vi "WPs and Obstacles 4.vi"(8 "Sim Robot Initial Long":dbl, 9 "Sim Robot Initial Lat":dbl, 11 "Real/Sim":bool) -> (0 "Obstacle Lats and Longs":cluster{"Obs Lats":dbl[], "Obs Longs":dbl[]} {"Obs Longs" format="%#_8g"; "Obs Lats" format="%#_8g"}, 1 "WP Lats and Longs":cluster{"WP Lats":dbl[], "WP Longs":dbl[]} {"WP Longs" format="%#_8g"; "WP Lats" format="%#_8g"}, 3 "WP Map":T1(graph))   [LabVIEW 2014]
panel:
  in  "Obstacle Real Longs":dbl[](array[numeric])=[81.2678, 81.267312, 81.267112, 81.267332, 81.267916, 81.267137, 81.267874, 81.267301, 81.267913, 81.26772] format="%#_8g"
  in  "Obstacle Real Lats":dbl[](array[numeric])=[37.1524, 37.152256, 37.152877, 37.152903, 37.152565, 37.152792, 37.152806, 37.152779, 37.152868, 37.152484] format="%#_8g"
  in  "WP Real Longs":dbl[](array[numeric])=[83.1954638, 83.19550076, 81.267112, 81.267332, 81.267916, 81.267137, 81.267874, 81.267301, 81.267913, 81.26772] format="%#_8g"
  in  "WP Real Lats":dbl[](array[numeric])=[42.678172477, 42.677950947, 37.152877, 37.152903, 37.152565, 37.152792, 37.152806, 37.152779, 37.152868, 37.152484] format="%#_8g"
  # "Waypoint and Obstacles 4 (Uses Paint)"
  # "Added Global sim painted map"
  # "Inputs:"
  # "20"
  # "12"
  # "Outputs:"
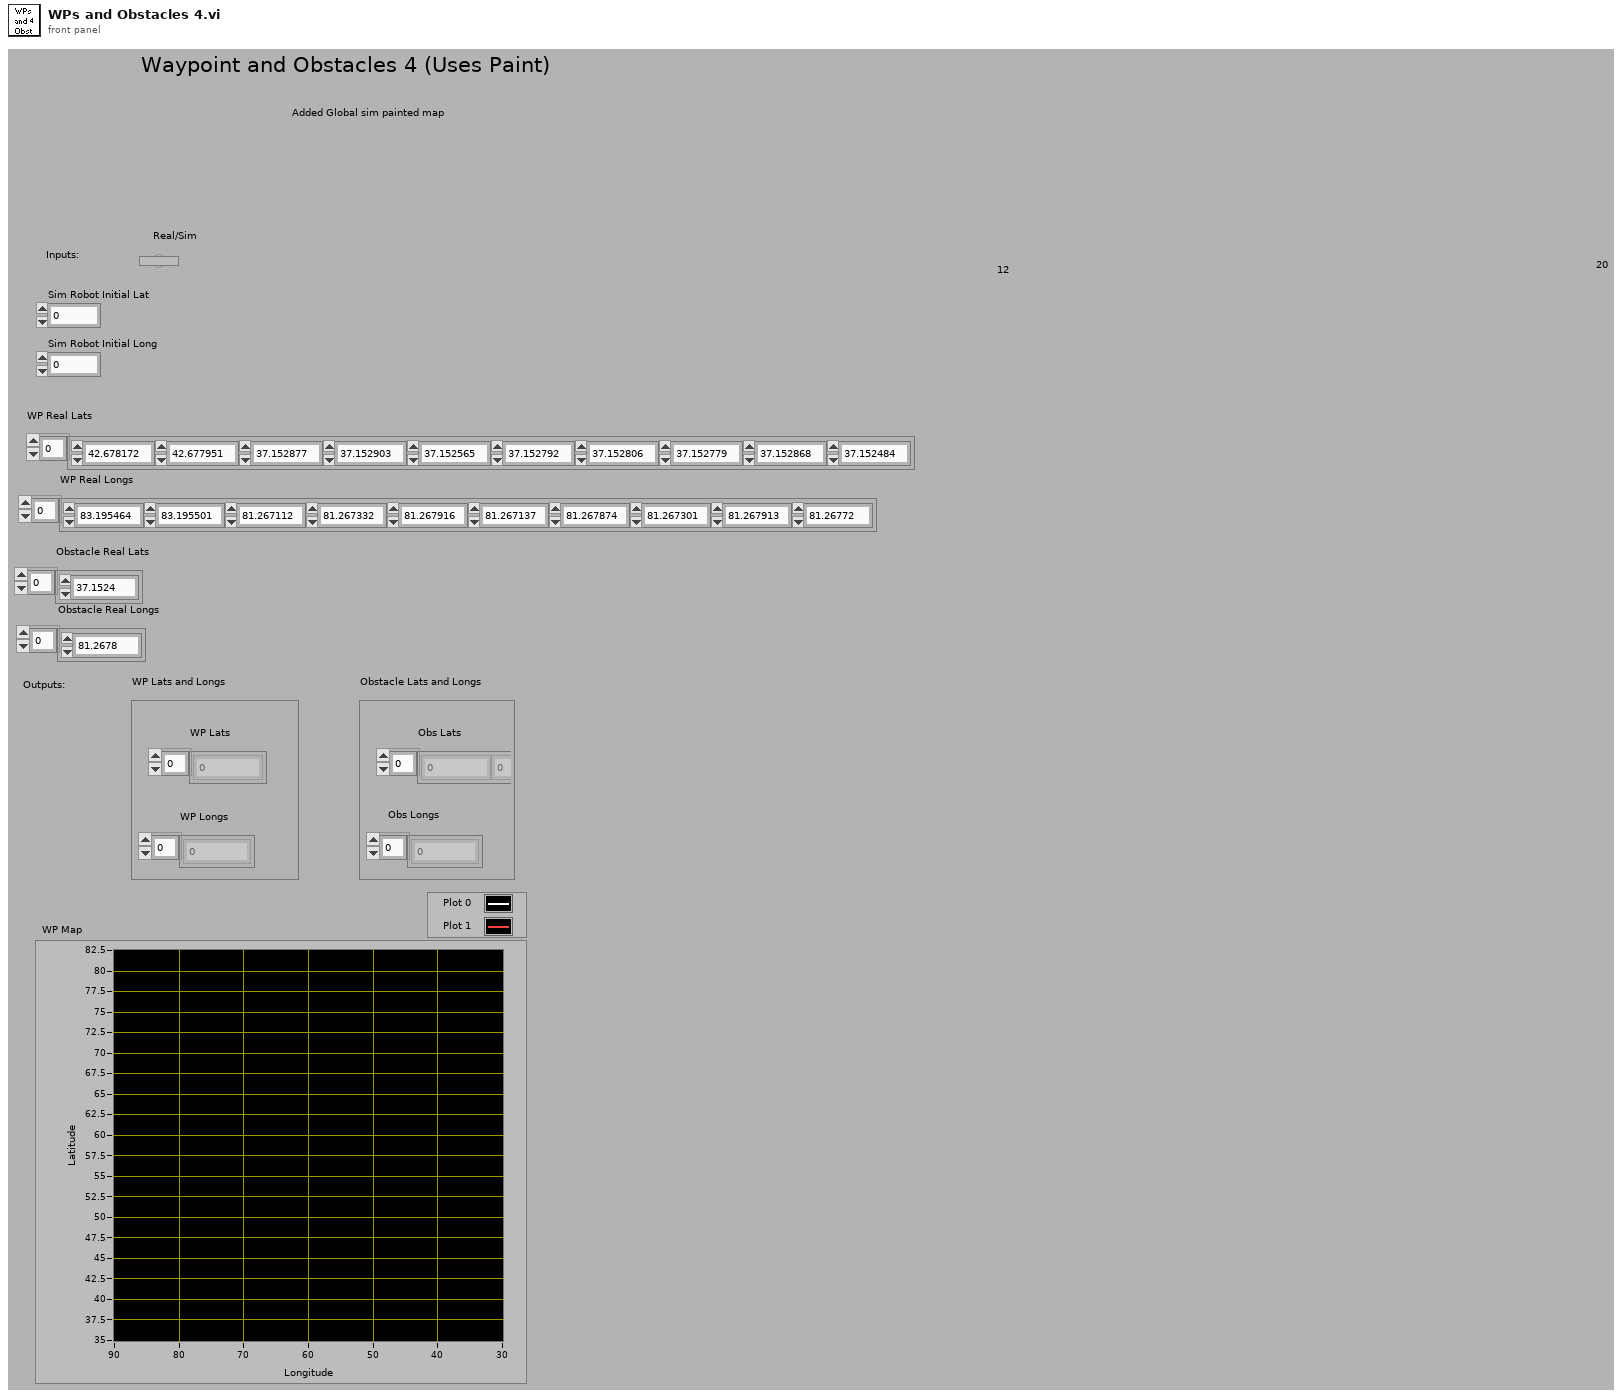
[diagram p1: front panel]
types:
  T1 = cluster{"Obstacle Longs":dbl[], "Obstacle Lats":dbl[]}[]
  T2 = cluster{"Obstacle Longs":dbl[], "Obstacle Lats":dbl[]}
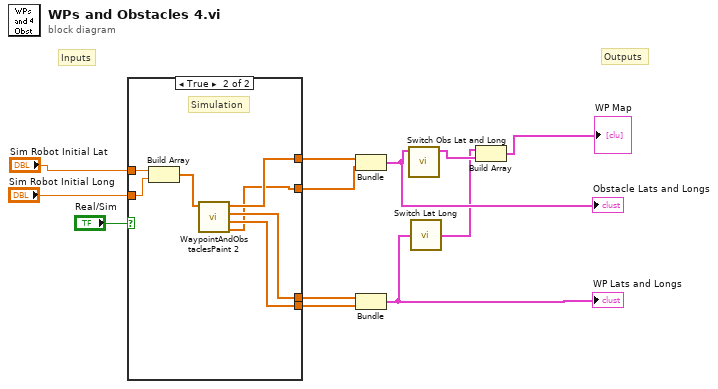
[diagram p0: block diagram]
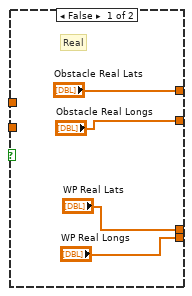
[diagram p2: hidden frame]
diagram:
  # "Inputs"
  # "Outputs"
  n1 = case shown="True" "Real/Sim" {
    tunnel: ["Obstacle Real Lats" w23] -> w11
    tunnel: ["Obstacle Real Longs" w17] -> w10
    tunnel: ["WP Real Lats" w19] -> w9
    tunnel: ["WP Real Longs" w18] -> w8
    tunnel: "Sim Robot Initial Lat" -> [_ w22]
    tunnel: "Sim Robot Initial Long" -> [_ w21]
    frame False {
      # "Real"
    }
    frame True {
      # "Simulation"
      n2 = Build Array(w22, w21) -> (w20:dbl[])
      n3 = call "WaypointAndObstaclesPaint 2.vi"("Simulated Initial Robot GPS Info:"=w20) -> ("Obs longs"=w17:dbl[], "WP Longs"=w18:dbl[], "WP Lats"=w19:dbl[], "Obs Lats"=w23:dbl[])  [unwired: 7 in]
    }
  }
  n4 = Bundle("Obs Lats"=w11, "Obs longs"=w10) -> (w6:cluster{"Obs Lats":dbl[], "Obs longs":dbl[]})  [unwired: 1 in]
  "Obstacle Lats and Longs" <- w6
  n5 = Bundle("WP Lats"=w9, "WP Longs"=w8) -> (w12:cluster{"WP Lats":dbl[], "WP Longs":dbl[]})  [unwired: 1 in]
  "WP Lats and Longs" <- w12
  n6 = call "Switch Obs Lat and Long.vi"("Obstacle Lats and Longs for GIC"=w6) -> ("Obstacle Lats and Longs switched"=w5:T2)  [unwired: 10 in]
  n7 = call "Switch Lat Long.vi"("WP Lats and Longs for GIC"=w12) -> ("WP Lats and Longs switched"=w4:cluster{"WP Longs":dbl[], "WP Lats":dbl[]})
  n8 = Build Array(w4, w5) -> (→"WP Map":T1)
